vi "Initialize Endpoint Configuration Page.vi"(8 "error in (no error)":errorcluster, 10 "Endpoint Configuration Page Controls":T1, 11 "Node Ptr":T2 format="%.0x") -> (0 "error out":errorcluster, 3 "Endpoint Configuration Section Ref out":T2 format="%.0x")   [LabVIEW 2017, in "SLSC Switch System Explorer.lvlib"]
uses:
  SLSC Switch System Explorer.lvlib
  <vilib>/NI Veristand/Custom Device API/Custom Device Item Ref.ctl
  Endpoint Configuration Page Controls.ctl
  Shared/UI Common/Sort Button.ctl
  Scripting/SLSC Switch Scripting.lvlib
  <vilib>/NI Veristand/Custom Device API/Custom Device API.lvlib
  Shared/UI Common/UI Common.lvlib
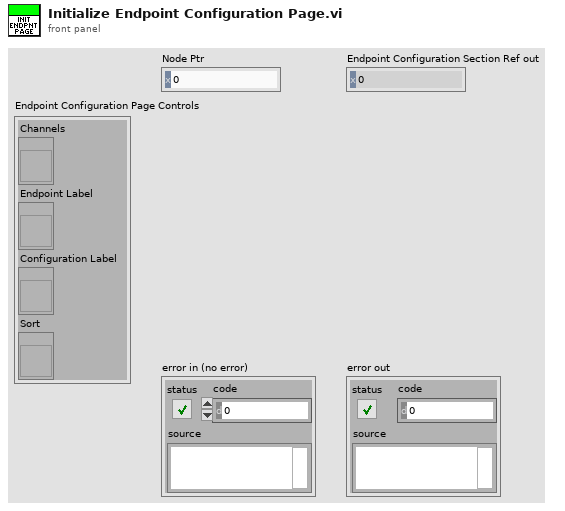
[diagram p1: front panel]
types:
  T1 = typedef "SLSC Switch System Explorer.lvlib/Endpoint Configuration Page Controls.ctl" = cluster{"Channels":refnum<vi>, "Endpoint Label":refnum<vi>, "Configuration Label":refnum<vi>, "Sort":refnum<vi>}
  T2 = typedef "Custom Device API.lvlib/Custom Device Item Ref.ctl" = u64
  T3 = enum8{"Enabled", "Disabled", "Disabled and Grayed Out"}
  T4 = typedef "SLSC Switch Shared.lvlib/Endpoint Configuration Cluster.ctl" = cluster{"Endpoint":string, "Configuration":T5}
  T5 = typedef "SLSC Switch Shared.lvlib/Endpoint Configuration Enum.ctl" = enum16{"Load", "Source", "Configuration"}
  T6 = typedef "SLSC Switch System Explorer.lvlib/Channel.ctl" = cluster{"Endpoint":string, "Configuration":T7}
  T7 = typedef "SLSC Switch System Explorer.lvlib/Channel Type.ctl" = enum16{"Load (Default)", "Source", "Configuration"}
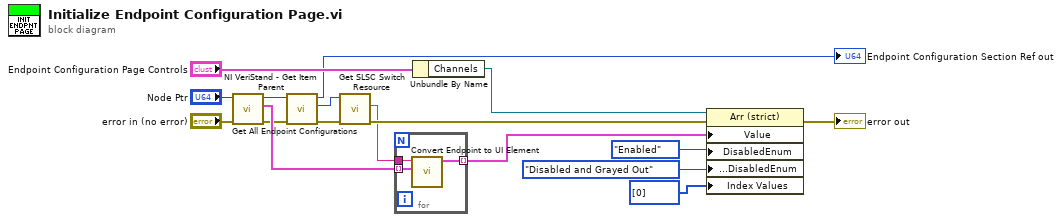
[diagram p0: block diagram]
diagram:
  n1 = call "Get All Endpoint Configurations.vi"("error in (no error)"="error in (no error)", "Endpoint Configuration Section Ref in"="Node Ptr") -> ("error out"=w8:errorcluster, "All Endpoint Configurations"=w17:T4[], "Endpoint Configuration Section Ref out"=w7:T2)  [unwired: 7 in]
  n2 = call <vilib>:"NI VeriStand - Get Item Parent.vi"("error in (no error)"=w8, "Item Ref in"=w7) -> ("error out"=w5:errorcluster, "Parent Ref"=w4:T2, "Item Ref out"=→"Endpoint Configuration Section Ref out":T2)  [unwired: 6 in, 1 out]
  n3 = call "Get SLSC Switch Resource.vi"("error in (no error)"=w5, "SLSC Switch Custom Device Ref in"=w4) -> ("error out"=w3:errorcluster, "Resource"=w2:string)  [unwired: 7 in, 1 out]
  n4 = for {
    tunnel: w17 -> [w18] mode=indexing
    tunnel: [w20] -> w11 mode=indexing
    tunnel: w2 -> [w19]
    n5 = call "Convert Endpoint to UI Element.vi"("Connection"=w18, "Resource"=w19) -> ("Channel"=w20:T6)  [unwired: 9 in]
  }
  n6 = Unbundle By Name("Endpoint Configuration Page Controls") -> ("Channels"=w13:refnum<vi>)
  n7 = property class="Arr (strict)"(reference=w13, error in=w3, "Value"=w11, "DisabledEnum"=T3."Enabled" ("Disabled"), "Array Element.DisabledEnum"=T3."Disabled and Grayed Out" ("Array Element.Disabled"), "Index Values"=u32[] [0]) -> (error out=→"error out":errorcluster)  [unwired: 1 out]
